vi "查询温度风扇.vi"(8 "error in (no error)":errorcluster, 11 "TCP Network Connection in":refnum<k5>) -> (0 "error out":errorcluster, 3 "TCP Network Connection out":refnum<k5>)   [LabVIEW 2015]
uses:
  Global/SeverGlobal.vi
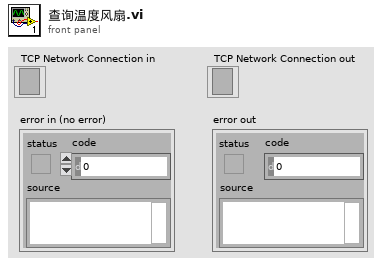
[diagram p1: front panel]
types:
  T1 = enum16{"Standard", "Buffered", "CRLF", "Immediate"}
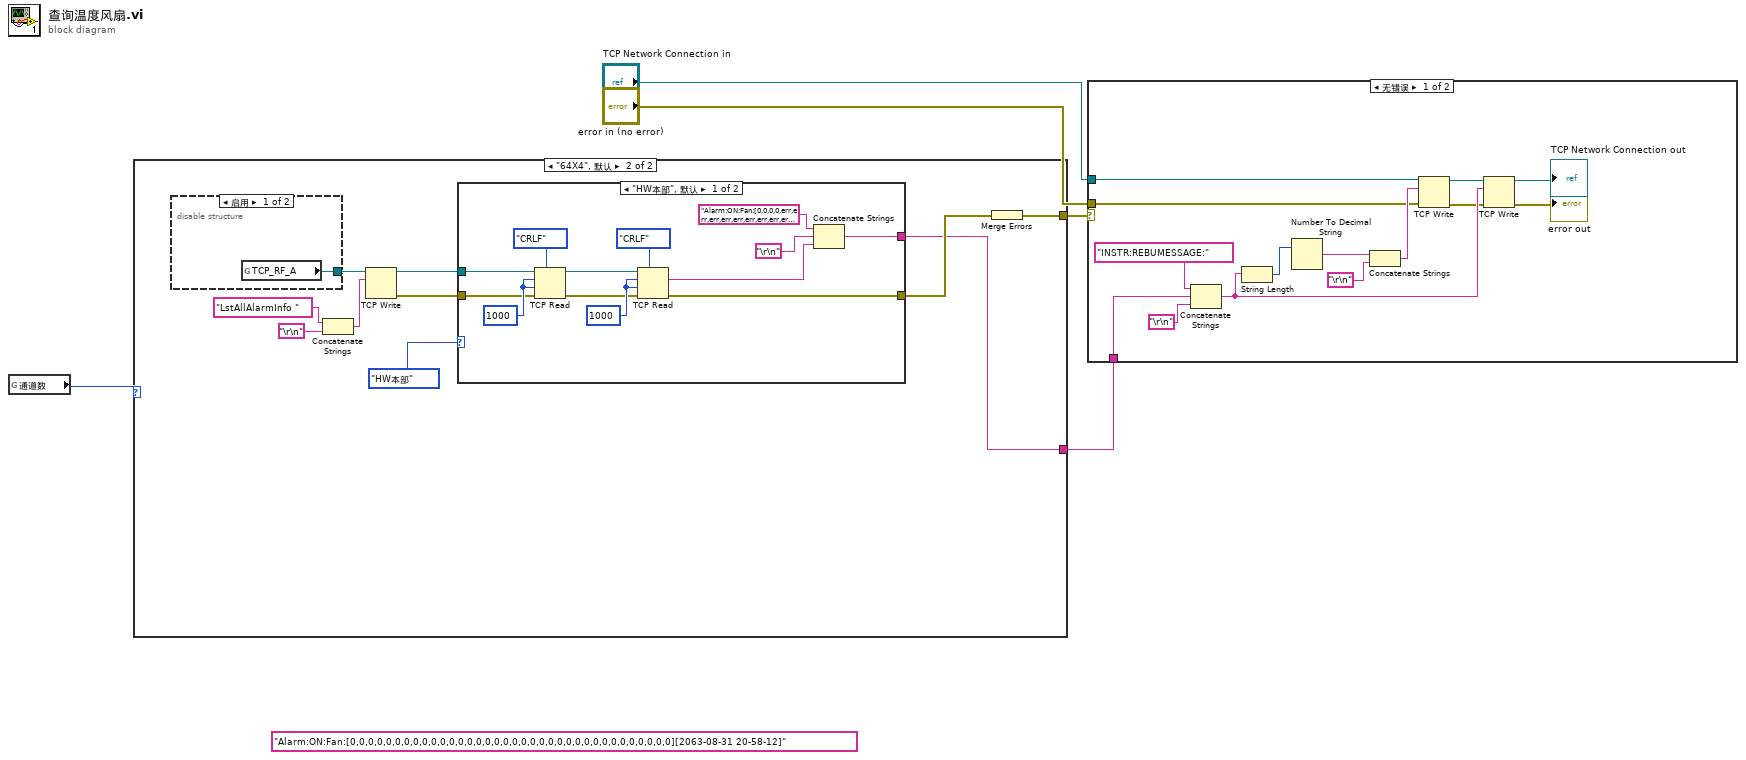
[diagram p0: block diagram]
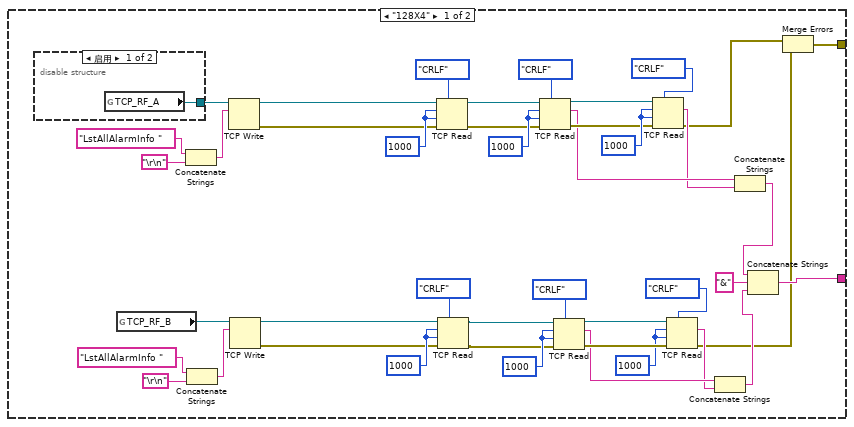
[diagram p2: hidden frame]
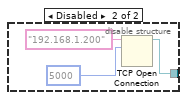
[diagram p3: hidden frame]
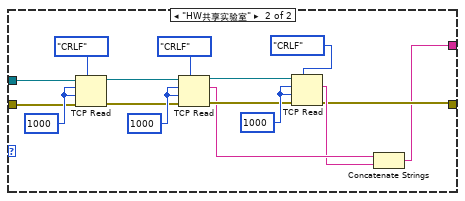
[diagram p4: hidden frame]
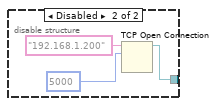
[diagram p5: hidden frame]
diagram:
  (unwired) "Alarm:ON:Fan:[0,0,0,0,0,0,0,0,0,0,0,0,0,0,0,0,0,0,0,0,0,0,0,0,0,0,0,0,0,0,0,0,0,0,0,0][2063-08-31 20-58-12]" ("字符串")
  n1 = global read "SeverGlobal.vi" "通道数"() -> (w1:enum16{"64X4", "128X4"})
  n2 = case shown="\"64X4\", 默认" w1 {
    tunnel: [w14 w54] -> w3
    tunnel: [w6 w62] -> w2
    frame "128X4" {
      w22 = 1000 ("timeout ms (25000)")
      w21 = 1000 ("timeout ms (25000)")
      w31 = 1000 ("timeout ms (25000)")
      w34 = 1000 ("timeout ms (25000)")
      w42 = 1000 ("timeout ms (25000)")
      w41 = 1000 ("timeout ms (25000)")
      n3 = disable-structure shown="启用" {
        disable-tunnel: [w49 w50] -> w36
        frame Enabled {
          n4 = global read "SeverGlobal.vi" "TCP_RF_A"() -> (w49:refnum<k5>)
        }
        frame Disabled {
          n5 = TCP Open Connection(address="192.168.1.200", remote port or service name=u16 5000) -> (connection ID=w50:refnum<k5>)  [unwired: 3 in, 1 out]
        }
      }
      n6 = global read "SeverGlobal.vi" "TCP_RF_B"() -> (w47:refnum<k5>)
      n7 = Concatenate Strings("LstAllAlarmInfo " ("元素"), "\r\n") -> (w39:string)
      n8 = Concatenate Strings("LstAllAlarmInfo " ("元素"), "\r\n") -> (w44:string)
      n9 = TCP Write(connection ID=w36, data in=w39) -> (connection ID out=w12:refnum<k5>, error out=w11:errorcluster)  [unwired: 2 in, 1 out]
      n10 = TCP Write(connection ID=w47, data in=w44) -> (connection ID out=w10:refnum<k5>, error out=w9:errorcluster)  [unwired: 2 in, 1 out]
      n11 = TCP Read(connection ID=w12, bytes to read=w41, error in (no error)=w11, 7:T1."CRLF" ("mode (standard)"), 9:w41) -> (connection ID out=w33:refnum<k5>, error out=w32:errorcluster)  [unwired: 1 out]
      n12 = TCP Read(connection ID=w10, bytes to read=w42, error in (no error)=w9, 7:T1."CRLF" ("mode (standard)"), 9:w42) -> (connection ID out=w19:refnum<k5>, error out=w18:errorcluster)  [unwired: 1 out]
      n13 = TCP Read(connection ID=w33, bytes to read=w34, error in (no error)=w32, 7:T1."CRLF" ("mode (standard)"), 9:w34) -> (connection ID out=w30:refnum<k5>, data out=w27:string, error out=w29:errorcluster)
      n14 = TCP Read(connection ID=w19, bytes to read=w21, error in (no error)=w18, 7:T1."CRLF" ("mode (standard)"), 9:w21) -> (connection ID out=w23:refnum<k5>, data out=w17:string, error out=w24:errorcluster)
      n15 = TCP Read(connection ID=w30, bytes to read=w31, error in (no error)=w29, 7:T1."CRLF" ("mode (standard)"), 9:w31) -> (data out=w25:string, error out=w8:errorcluster)  [unwired: 1 out]
      n16 = TCP Read(connection ID=w23, bytes to read=w22, error in (no error)=w24, 7:T1."CRLF" ("mode (standard)"), 9:w22) -> (data out=w16:string, error out=w7:errorcluster)  [unwired: 1 out]
      n17 = Concatenate Strings(w17, w16) -> (w15:string)
      n18 = Concatenate Strings(w27, w25) -> (w26:string)
      n19 = Concatenate Strings(w26, "&" ("string"), w15) -> (w14:string)
      n20 = Merge Errors(w8, w7) -> (w6:errorcluster)
    }
    frame "64X4", Default {
      n21 = disable-structure shown="启用" {
        disable-tunnel: [w92 w93] -> w58
        frame Enabled {
          n22 = global read "SeverGlobal.vi" "TCP_RF_A"() -> (w92:refnum<k5>)
        }
        frame Disabled {
          n23 = TCP Open Connection(address="192.168.1.200", remote port or service name=u16 5000) -> (connection ID=w93:refnum<k5>)  [unwired: 3 in, 1 out]
        }
      }
      n24 = Concatenate Strings("LstAllAlarmInfo " ("元素"), "\r\n") -> (w61:string)
      n25 = TCP Write(connection ID=w58, data in=w61) -> (connection ID out=w57:refnum<k5>, error out=w56:errorcluster)  [unwired: 2 in, 1 out]
      n26 = case shown="\"HW本部\", 默认" enum16{"HW本部", "HW共享实验室"}."HW本部" {
        tunnel: w57 -> [w69 w79]
        tunnel: w56 -> [w68 w78]
        tunnel: [w64 w77] -> w55
        tunnel: [w63 w76] -> w54
        frame "HW本部", Default {
          w72 = 1000 ("timeout ms (25000)")
          w75 = 1000 ("timeout ms (25000)")
          n27 = TCP Read(connection ID=w69, bytes to read=w75, error in (no error)=w68, 7:T1."CRLF" ("mode (standard)"), 9:w75) -> (connection ID out=w71:refnum<k5>, error out=w70:errorcluster)  [unwired: 1 out]
          n28 = TCP Read(connection ID=w71, bytes to read=w72, error in (no error)=w70, 7:T1."CRLF" ("mode (standard)"), 9:w72) -> (data out=w65:string, error out=w64:errorcluster)  [unwired: 1 out]
          n29 = Concatenate Strings("Alarm:ON:Fan:[0,0,0,0,err,err,err,err,err,err,err,err,err,err,err,err,err,err,err,err,err,err,err,err,err,err,err,err,err,err,err,err,0,0,0,0][2015-10-11 16-29-58]" ("元素"), "\r\n", w65) -> (w63:string)
        }
        frame "HW共享实验室" {
          w85 = 1000 ("timeout ms (25000)")
          w88 = 1000 ("timeout ms (25000)")
          w91 = 1000 ("timeout ms (25000)")
          n30 = TCP Read(connection ID=w79, bytes to read=w91, error in (no error)=w78, 7:T1."CRLF" ("mode (standard)"), 9:w91) -> (connection ID out=w87:refnum<k5>, error out=w86:errorcluster)  [unwired: 1 out]
          n31 = TCP Read(connection ID=w87, bytes to read=w88, error in (no error)=w86, 7:T1."CRLF" ("mode (standard)"), 9:w88) -> (connection ID out=w84:refnum<k5>, data out=w81:string, error out=w83:errorcluster)
          n32 = TCP Read(connection ID=w84, bytes to read=w85, error in (no error)=w83, 7:T1."CRLF" ("mode (standard)"), 9:w85) -> (data out=w80:string, error out=w77:errorcluster)  [unwired: 1 out]
          n33 = Concatenate Strings(w81, w80) -> (w76:string)
        }
      }
      n34 = Merge Errors(w55) -> (w62:errorcluster)
    }
  }
  n35 = case shown="无错误" w2 {
    tunnel: "error in (no error)" -> [w103 _]
    tunnel: "TCP Network Connection in" -> [w101 _]
    tunnel: w3 -> [w96 _]
    frame No Error {
      n36 = Concatenate Strings("INSTR:REBUMESSAGE:", w96, "\r\n") -> (w105:string)
      n37 = String Length(string=w105) -> (length=w106:i32)
      n38 = Number To Decimal String(number=w106) -> (decimal integer string=w108:string)  [unwired: 1 in]
      n39 = Concatenate Strings(w108, "\r\n") -> (w109:string)
      n40 = TCP Write(connection ID=w101, data in=w109, error in (no error)=w103) -> (connection ID out=w102:refnum<k5>, error out=w104:errorcluster)  [unwired: 1 in, 1 out]
      n41 = TCP Write(connection ID=w102, data in=w105, error in (no error)=w104) -> (connection ID out=→"TCP Network Connection out":refnum<k5>, error out=→"error out":errorcluster)  [unwired: 1 in, 1 out]
    }
    frame Error {
    }
  }
